vi "Set TWM Measurement.vi"(4 "status ref (none)":refnum<vi>, 5 "Loop iteration":i32, 7 "Measurement properties":T1={"Measurement frequencies (Hz)"=[], "Sampling frequency (Hz)"=1.0, "Signal amplitude (V)"=50.0, "AC-DC settle time (s)"=50.0, "Record length (multiples of period)"=[], "Measurement template file"=path "", "Row of START keyword"=0, "Row of STOP keyword"=0} {"Record length (multiples of period)" format="%#_3p"; "Sampling frequency (Hz)" format="%#_3p"; "Measurement frequencies (Hz)" format="%#_3p"}, 8 "error in":errorcluster, 11 "handle":i32) -> (0 "error out":errorcluster, 3 "handle out":i32)   [LabVIEW 2020]
uses:
  external libraries/TWM-1.8.7.0-client/TWM Client.lvlib
  external libraries/TWM-1.8.7.0-client/infolib.lvlib
  external libraries/TWM-1.8.7.0-client/I64.vi
  external libraries/TWM-1.8.7.0-client/EXT.vi
  external libraries/TWM-1.8.7.0-client/String.vi
  Type definitions/Measuement properties.ctl
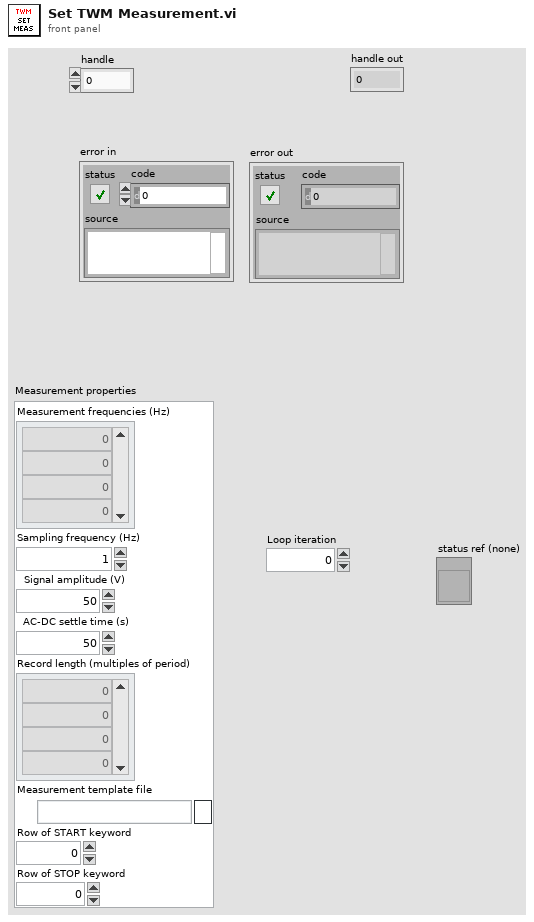
[diagram p1: front panel]
types:
  T1 = typedef "Measuement properties.ctl" = cluster{"Measurement frequencies (Hz)":dbl[], "Sampling frequency (Hz)":dbl, "Signal amplitude (V)":dbl, "AC-DC settle time (s)":dbl, "Record length (multiples of period)":dbl[], "Measurement template file":path, "Row of START keyword":i32, "Row of STOP keyword":i32}
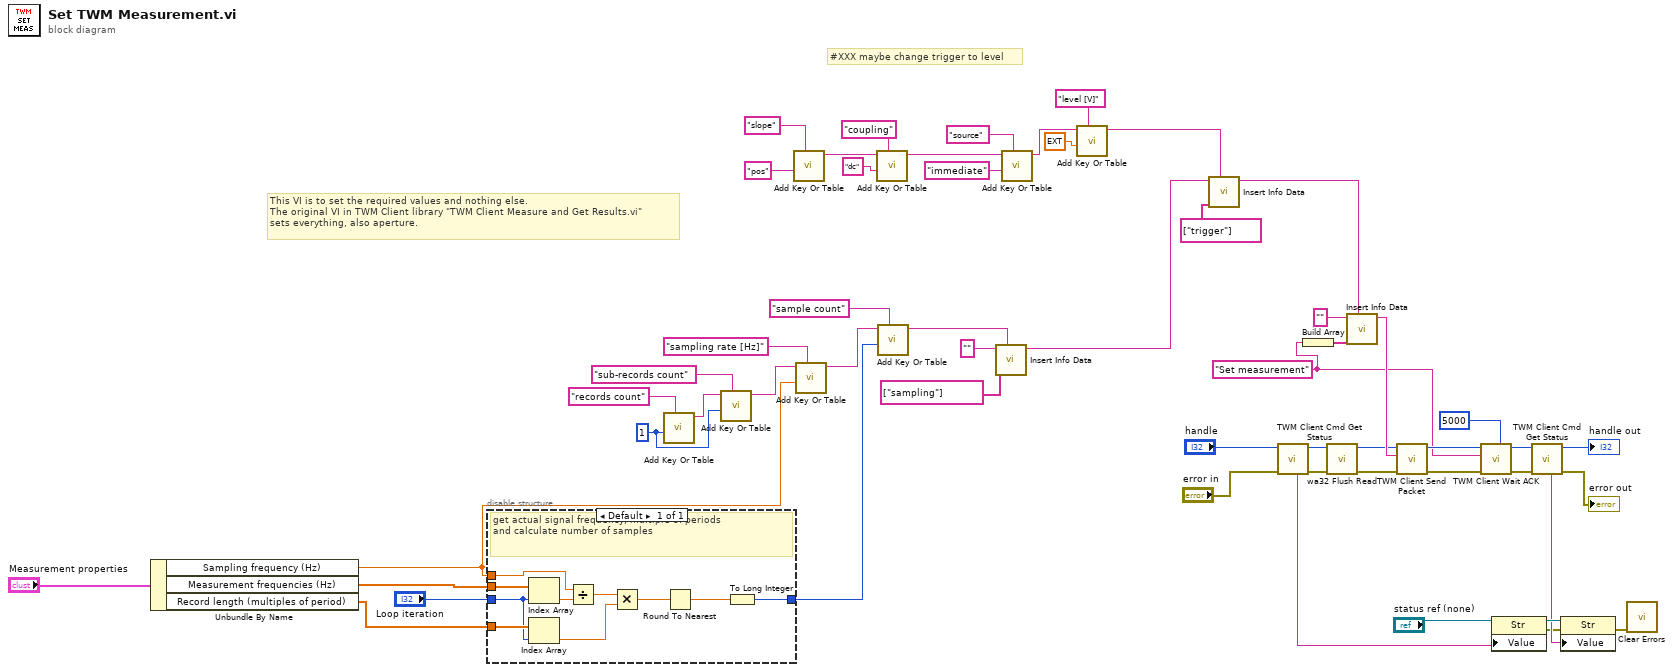
[diagram p0: block diagram]
diagram:
  w40 = 1 ("sub-records")
  w49 = "Set measurement" ("section name")
  # "#XXX maybe change trigger to level"
  # "This VI is to set the required values and nothing else.\nThe original VI in TWM Client library \"TWM Client Measure and Get Results.vi\"\nsets everything, also aperture."
  n1 = Unbundle By Name("Measurement properties") -> ("Sampling frequency (Hz)"=w2:dbl, "Measurement frequencies (Hz)"=w5:dbl[], "Record length (multiples of period)"=w4:dbl[])
  n2 = disable-structure shown="Default" {
    disable-tunnel: w5 -> [w65]
    disable-tunnel: w4 -> [w64]
    disable-tunnel: "Loop iteration" -> [w63]
    disable-tunnel: w2 -> [w62]
    disable-tunnel: [w56] -> w1
    frame Enabled {
      # "get actual signal frequency, multiple of periods\nand calculate number of samples"
      n3 = Index Array(array=w65, index=w63) -> (element=w61:dbl)
      n4 = Index Array(array=w64, index=w63) -> (element=w59:dbl)
      n5 = Divide(x=w62, y=w61) -> (x/y=w60:dbl)
      n6 = Multiply(x=w60, y=w59) -> (x*y=w58:dbl)
      n7 = Round To Nearest(number=w58) -> (nearest integer value=w57:dbl)
      n8 = To Long Integer(number=w57) -> (32bit integer=w56:i32)
    }
  }
  n9 = call-poly "Add Key Or Table.vi"("key description"="records count", "numeric"=w40) -> ("info data out"=w43:string)  [unwired: 8 in, 1 out]
  n10 = call-poly "Add Key Or Table.vi"("key description"="sub-records count", "numeric"=w40, "info data"=w43) -> ("info data out"=w38:string)  [unwired: 7 in, 1 out]
  n11 = call-poly "Add Key Or Table.vi"("key description"="slope", "string"="pos" ("key description")) -> ("info data out"=w22:string)  [unwired: 8 in, 1 out]
  n12 = call-poly "Add Key Or Table.vi"("key description"="sampling rate [Hz]", "numeric"=w2, "info data"=w38) -> ("info data out"=w37:string)  [unwired: 7 in, 1 out]
  n13 = call-poly "Add Key Or Table.vi"("key description"="coupling", "string"="dc" ("key description"), "info data"=w22) -> ("info data out"=w26:string)  [unwired: 7 in, 1 out]
  n14 = call-poly "Add Key Or Table.vi"("key description"="sample count", "numeric"=w1, "info data"=w37) -> ("info data out"=w36:string)  [unwired: 7 in, 1 out]
  n15 = call "Insert Info Data.vi"("info data to insert"=w36, "sections"=string[] ["sampling"], "info data"="") -> ("info data out"=w35:string)  [unwired: 7 in, 1 out]
  n16 = call-poly "Add Key Or Table.vi"("key description"="source", "string"="immediate" ("key description"), "info data"=w26) -> ("info data out"=w28:string)  [unwired: 7 in, 1 out]
  n17 = call-poly "Add Key Or Table.vi"("key description"="level [V]", "numeric"=ext 2.5, "info data"=w28) -> ("info data out"=w31:string)  [unwired: 7 in, 1 out]
  n18 = call "Insert Info Data.vi"("info data to insert"=w31, "sections"=string[] ["trigger"], "info data"=w35) -> ("info data out"=w34:string)  [unwired: 7 in, 1 out]
  n19 = call "TWM Client Cmd Get Status.vi"("error in"="error in", "handle"="handle") -> ("error out"=w9:errorcluster, "handle out"=w20:i32, "status string"=w18:string)  [unwired: 5 in, 2 out]
  n20 = Build Array(w49) -> (w54:string[])
  n21 = call "wa32 Flush Read.vi"("error in"=w9, "handle"=w20) -> ("error out"=w48:errorcluster, "handle out"=w47:i32)  [unwired: 7 in, 1 out]
  n22 = call "Insert Info Data.vi"("info data to insert"=w34, "sections"=w54, "info data"="") -> ("info data out"=w55:string)  [unwired: 7 in, 1 out]
  n23 = call "TWM Client Send Packet.vi"("error in"=w48, "command string"=w55, "handle"=w47) -> ("error out"=w52:errorcluster, "handle out"=w51:i32)  [unwired: 7 in]
  n24 = call "TWM Client Wait ACK.vi"("timeout [ms] (3000)"=5000 ("timeout [ms] (1000)"), "error in"=w52, "command header"=w49, "handle"=w51) -> ("error out"=w16:errorcluster, "handle out"=w15:i32)  [unwired: 6 in]
  n25 = property class="Str"(reference="status ref (none)", "Value"=w18) -> (reference out=w17:refnum<vi>, error out=w10:errorcluster)  [unwired: 1 in]
  n26 = call "TWM Client Cmd Get Status.vi"("error in"=w16, "handle"=w15) -> ("error out"=→"error out":errorcluster, "handle out"=→"handle out":i32, "status string"=w12:string)  [unwired: 5 in, 2 out]
  n27 = property class="Str"(reference=w17, error in=w10, "Value"=w12) -> (error out=w11:errorcluster)  [unwired: 1 out]
  n28 = call <vilib>:"Clear Errors.vi"("error in (no error)"=w11) -> ()  [unwired: 5 in, 2 out]
